vi "maintainAudioBuffer.vi"(8 "error in (no error)":errorcluster, 9 "Samples per\nacquisition chunk":i32, 10 "Audio buffer size (frames)":i32, 11 "Audio data queue in":refnum<queue>) -> (0 "error out":errorcluster)   [LabVIEW 2017]
doc: "Maintain the # of elements in the audio queue to be less than the desired buffer size."
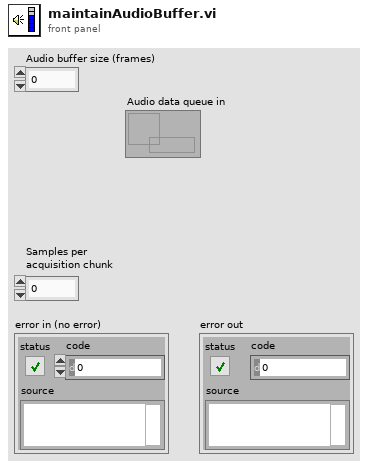
[diagram p1: front panel]
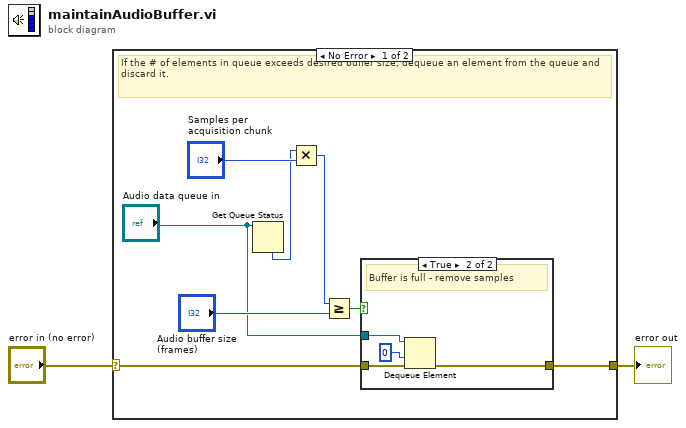
[diagram p0: block diagram]
diagram:
  n1 = case shown="No Error" "error in (no error)" {
    selector: "error in (no error)" -> [w5 w16]
    tunnel: [w6 w16] -> w2
    frame No Error {
      # "If the # of elements in queue exceeds desired buffer size, dequeue an element from the queue and discard it."
      n2 = Get Queue Status(queue="Audio data queue in") -> (# elements in queue=w4:i32)  [unwired: 2 in, 7 out]
      n3 = Multiply(x=w4, y="Samples per\nacquisition chunk") -> (x*y=w7:i32)
      n4 = Greater Or Equal?(x=w7, y="Audio buffer size (frames)") -> (x >= y?=w10:bool)
      n5 = case shown="True" w10 {
        tunnel: [w11 w14] -> w6
        tunnel: "Audio data queue in" -> [_ w13]
        tunnel: w5 -> [w11 w12]
        frame False {
          # "Buffer not full yet"
        }
        frame True {
          # "Buffer is full - remove samples"
          n6 = Dequeue Element(queue=w13, timeout in ms (-1)=0, error in (no error)=w12) -> (error out=w14:errorcluster)  [unwired: 3 out]
        }
      }
    }
    frame Error {
    }
  }
  "error out" <- w2
